vi "HTML_CreateTable.vi"(8 "Error In":errorcluster, 9 "Table body[2D]":string[][](array[string])=[["Airi Satou", "Tokyo", "33"], ["Caesar Vance", "New York", "21"], ["Sonya Frost", "Edinburgh", "23"]], 10 "Table head[2D]":string[][](array[string])=[["Name", "Office", "Age"]]) -> (0 "Error Out":errorcluster, 2 "resulting string":string)   [LabVIEW 2014]
panel:
  in  "Table css-Attributes[]":string[][](array[string])=[["width", "100%"]]
  in  "Table Classes[]":string[](array[string])=[""]
  in  "Table IDs[]":string[](array[string])=["example"]
  in  "compress?":bool
  in  "Table foot[2D]":string[][](array[string])=[["Name", "Office", "Age"]]
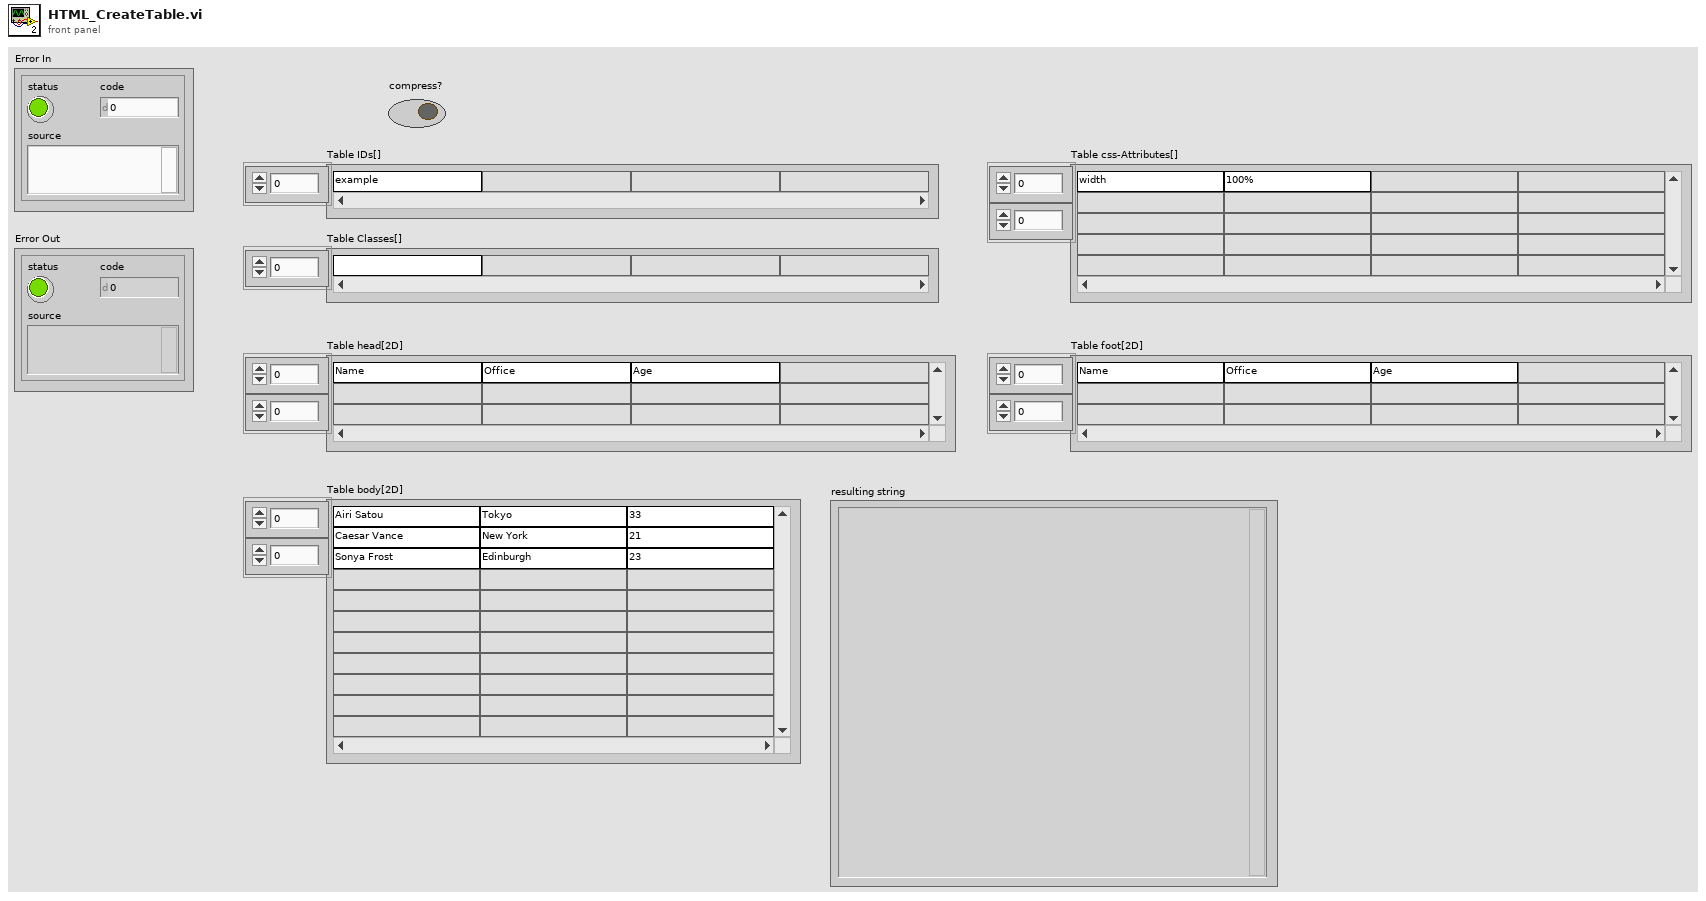
[diagram p1: front panel]
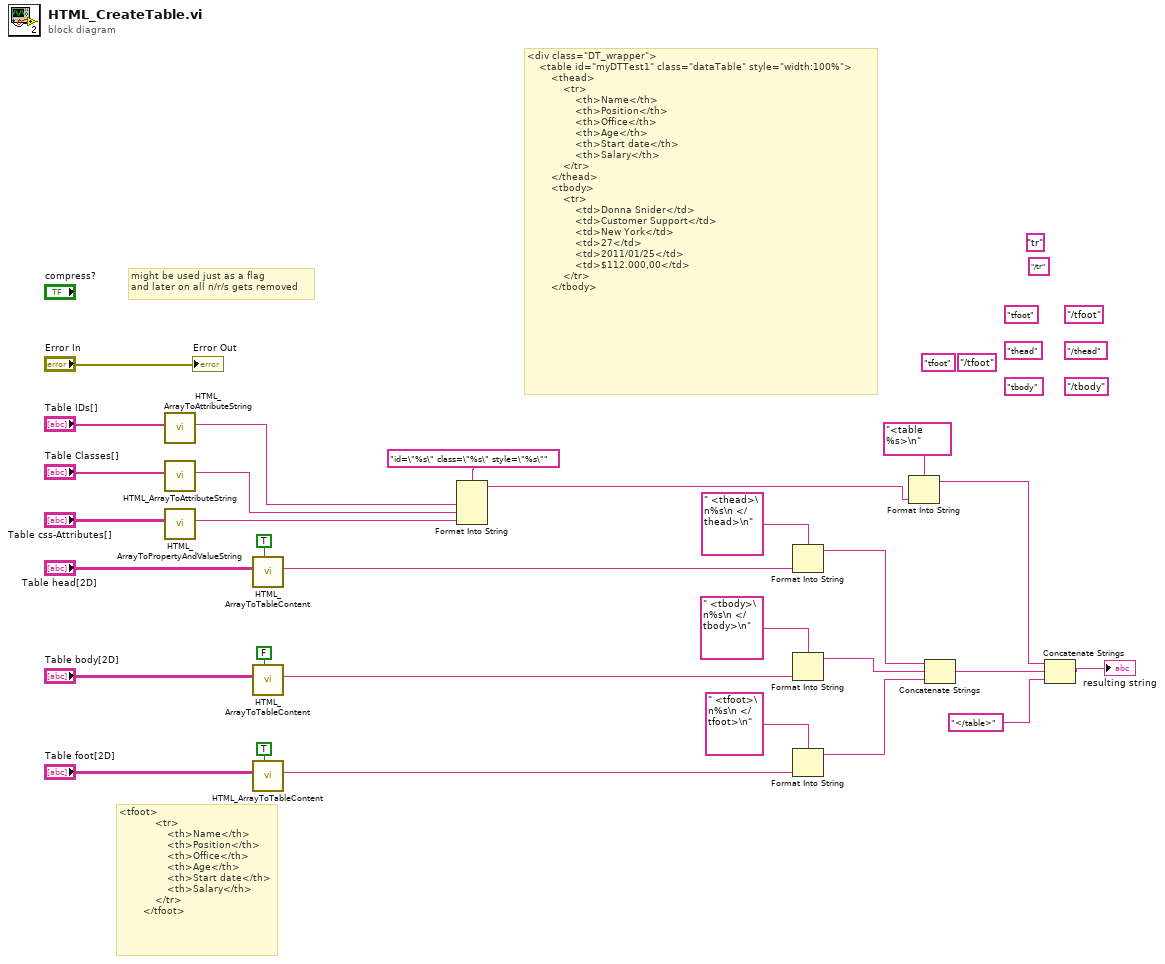
[diagram p0: block diagram]
diagram:
  (unwired) "/tfoot"
  (unwired) "tfoot"
  (unwired) "/tr"
  (unwired) "tr"
  (unwired) "/thead"
  (unwired) "/tbody"
  (unwired) "/tfoot"
  (unwired) "tbody"
  (unwired) "tfoot"
  (unwired) "thead"
  # "<tfoot>\n            <tr>\n                <th>Name</th>\n                <th>Position</th>\n                <th>Office</th>\n                <th>Age</th>\n                <th>Start date</th>\n                <th>Salary</th>\n            </tr>\n        </tfoot>"
  # "might be used just as a flag\nand later on all n/r/s gets removed"
  # "<div class=\"DT_wrapper\">\n    <table id=\"myDTTest1\" class=\"dataTable\" style=\"width:100%\">\n        <thead>\n            <tr>\n                <th>Name</th>\n                <th>Position</th>\n                <th>Office</th>\n                <th>Age</th>\n                <th>Start date</th>\n                <th>Salary</th>\n            </tr>\n        </thead>\n        <tbody>\n            <tr>\n                <td>Donna Snider</td>\n                <td>Customer Support</td>\n                <td>New York</td>\n                <td>27</td>\n                <td>2011/01/25</td>\n                <td>$112.000,00</td>\n            </tr>\n        </tbody>"
  n1 = call "HTML_ArrayToAttributeString.vi"("Attribute List[]"="Table IDs[]") -> ("spreadsheet string"=w17:string)  [unwired: 10 in]
  n2 = call "HTML_ArrayToAttributeString.vi"("Attribute List[]"="Table Classes[]") -> ("spreadsheet string"=w15:string)  [unwired: 10 in]
  n3 = call "HTML_ArrayToPropertyAndValueString.vi"("Table css-Attributes[]"="Table css-Attributes[]") -> ("spreadsheet string"=w13:string)  [unwired: 10 in]
  n4 = call "HTML_ArrayToTableContent.vi"("<th> (T) / <td> (F)"=TRUE, "Table foot[2D]"="Table head[2D]") -> ("resulting string"=w10:string)  [unwired: 9 in]
  n5 = call "HTML_ArrayToTableContent.vi"("<th> (T) / <td> (F)"=FALSE, "Table foot[2D]"="Table body[2D]") -> ("resulting string"=w5:string)  [unwired: 9 in]
  n6 = call "HTML_ArrayToTableContent.vi"("<th> (T) / <td> (F)"=TRUE, "Table foot[2D]"="Table foot[2D]") -> ("resulting string"=w4:string)  [unwired: 9 in]
  n7 = Format Into String(format string="id=\"%s\" class=\"%s\" style=\"%s\"", w17, w15, w13) -> (resulting string=w23:string)  [unwired: 2 in, 1 out]
  n8 = Format Into String(format string=" <thead>\n%s\n </thead>\n", w10) -> (resulting string=w11:string)  [unwired: 2 in, 1 out]
  n9 = Format Into String(format string=" <tbody>\n%s\n </tbody>\n", w5) -> (resulting string=w25:string)  [unwired: 2 in, 1 out]
  n10 = Format Into String(format string=" <tfoot>\n%s\n </tfoot>\n", w4) -> (resulting string=w3:string)  [unwired: 2 in, 1 out]
  n11 = Format Into String(format string="<table %s>\n", w23) -> (resulting string=w22:string)  [unwired: 2 in, 1 out]
  n12 = Concatenate Strings(w11, w25, w3) -> (w21:string)
  n13 = Concatenate Strings(w22, w21, "</table>") -> (→"resulting string":string)
  "Error Out" <- "Error In"
